vi "Msg.vi"(7 "jettl in":refnum<class "jettl.lvclass">, 11 "xxxxx Msg Strategy in":refnum<class "xxxxx Msg Strategy.lvclass">) -> (5 "jettl out":refnum<class "jettl.lvclass">)   [LabVIEW 2021, in "jettl Tools.lvlib" / "jettl Msg xxxxx.lvlib" / "xxxxx Msg Strategy.lvclass"]
uses:
  xxxxx Msg Strategy.lvclass
  jettl/jettl/jettl.lvclass
  xxxxx/xxxxx.lvclass
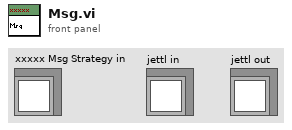
[diagram p1: front panel]
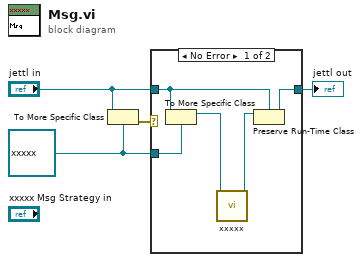
[diagram p0: block diagram]
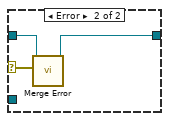
[diagram p2: hidden frame]
diagram:
  w1 = refnum<class "xxxxx.lvclass"> refnum ("Providers.lvlib:jettl Msg xxxxx.lvlib:xxxxx.lvclass")
  n1 = To More Specific Class(target class=w1, reference="jettl in") -> (error out=w4:errorcluster)  [unwired: 1 in, 1 out]
  n2 = case shown="No Error" w4 {
    selector: w4 -> [_ w11]
    tunnel: [w7 w10] -> w2
    tunnel: "jettl in" -> [w8 w12]
    tunnel: w1 -> [w9 _]
    frame No Error {
      n3 = To More Specific Class(target class=w9, reference=w8) -> (specific class reference=w6:refnum<class "xxxxx.lvclass">)  [unwired: 1 in, 1 out]
      n4 = call-dynamic "xxxxx.vi"("xxxxx in"=w6) -> ("xxxxx out"=w5:refnum<class "xxxxx.lvclass">)  [unwired: 10 in]
      n5 = Preserve Run-Time Class(object in=w5, 2:w8) -> (object out=w7:refnum<class "jettl.lvclass">)  [unwired: 1 in, 1 out]
    }
    frame Error {
      n6 = call-dynamic "Merge Error.vi"("Error"=w11, "Merge Error in"=w12) -> ("Merge Error out"=w10:refnum<class "jettl.lvclass">)  [unwired: 9 in]
    }
  }
  "jettl out" <- w2
